vi "Save File Create Runtime File Change.vi"(8 "Error In":errorcluster, 11 "Root Folder Path":path) -> (0 "Error Out":errorcluster, 3 "File Number String":string="0")   [LabVIEW 2018, in "Save File.lvlib"]
uses:
  Save File.lvlib
panel:
  out "filenames":string[](array[string])
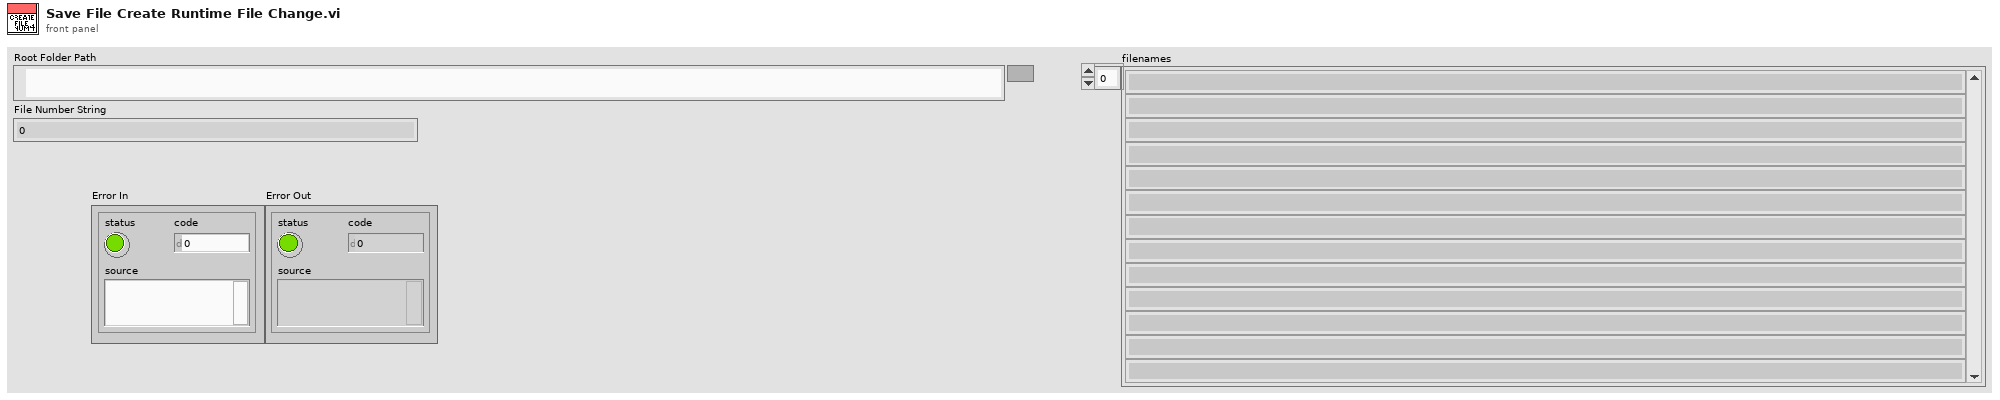
[diagram p1: front panel]
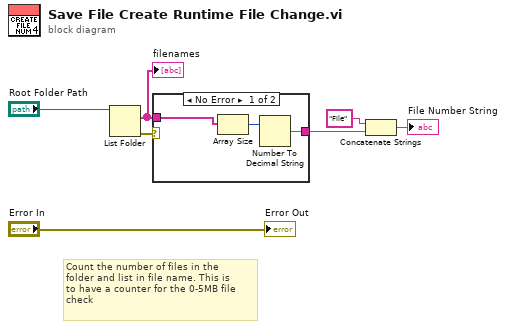
[diagram p0: block diagram]
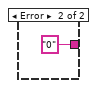
[diagram p2: hidden frame]
diagram:
  # "Count the number of files in the \nfolder and list in file name. This is \nto have a counter for the 0-5MB file \ncheck"
  n1 = List Folder(path="Root Folder Path") -> (filenames=w6:string[], error out=w5:errorcluster)  [unwired: 3 in, 2 out]
  "filenames" <- w6
  n2 = case shown="No Error" w5 {
    tunnel: w6 -> [w9 _]
    tunnel: [w8 "0"] -> w3
    frame No Error {
      n3 = Array Size(array=w9) -> (size(s)=w10:i32)
      n4 = Number To Decimal String(number=w10) -> (decimal integer string=w8:string)  [unwired: 1 in]
    }
    frame Error {
    }
  }
  n5 = Concatenate Strings("File" ("string"), w3) -> (→"File Number String":string)
  "Error Out" <- "Error In"
